vi "wmlf Defects Script.vi"(0 "File Path":path, 2 "threshoulds":dbl[](array[numeric])=[900.0, 900.0, 1000.0, 1200.0, 1800.0, 1800.0, 2000.0, 2400.0], 3 "margin":dbl[](array[numeric]), 5 "Image 3":T1(plugin-control), 7 "error in (no error)":errorcluster) -> (18 "function return":i32, 20 "x-y defects locs":dbl[][](array[numeric]), 21 "defnum":dbl, 22 "def type":dbl, 23 "frame situation":dbl, 24 "obj num":dbl, 25 "def ratio":dbl, 26 "crop array":dbl[][](array[numeric]), 27 "error out":errorcluster)   [LabVIEW 2019, in "defectsWrapper.lvlib"]
doc: "int wmlfDefectsScript(double* c2dArray, double* d2dArray, double* e2dArray ,double* f2dArray, double* g2dArray,\n double* h2dArray , double* i2dArray, double* j2dArray,double* k2dArray, double* l2dArray, int numRows, int numColumns,\n int Rows, int Columns, int Rows1, int Columns1, int Rows2, int Columns2, int Rows3, int Columns3,\n int Rows4, int Columns4,int Rows5, int Columns5,int Rows6, int Columns6, int Rows7, int Columns7,\n int Rows8, int Columns8 );"
uses:
  defectsWrapper.lvlib
  defectsWrapper.dll
panel:
  out "x array":dbl[](array[numeric])
  out "ydef":dbl[][](array[numeric])
  out "xdef":dbl[][](array[numeric])
  out "initialized array":dbl[][](array[numeric])
  out "Image 2":T1(plugin-control)
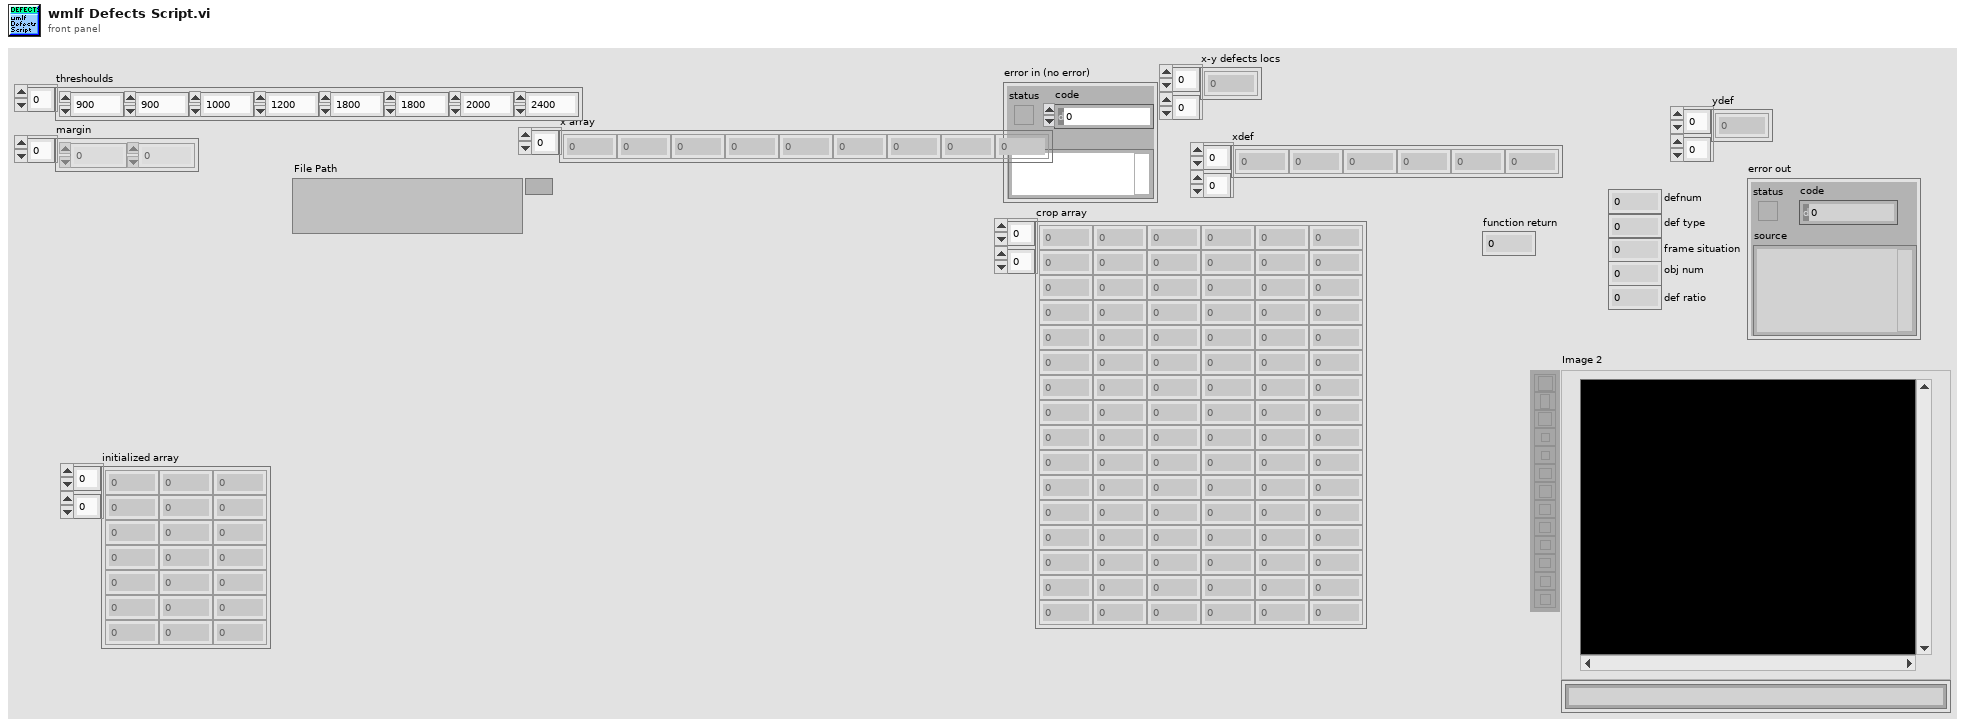
[diagram p1: front panel]
types:
  T1 = typedef "IMAQ Image.ctl" = refnum<image>
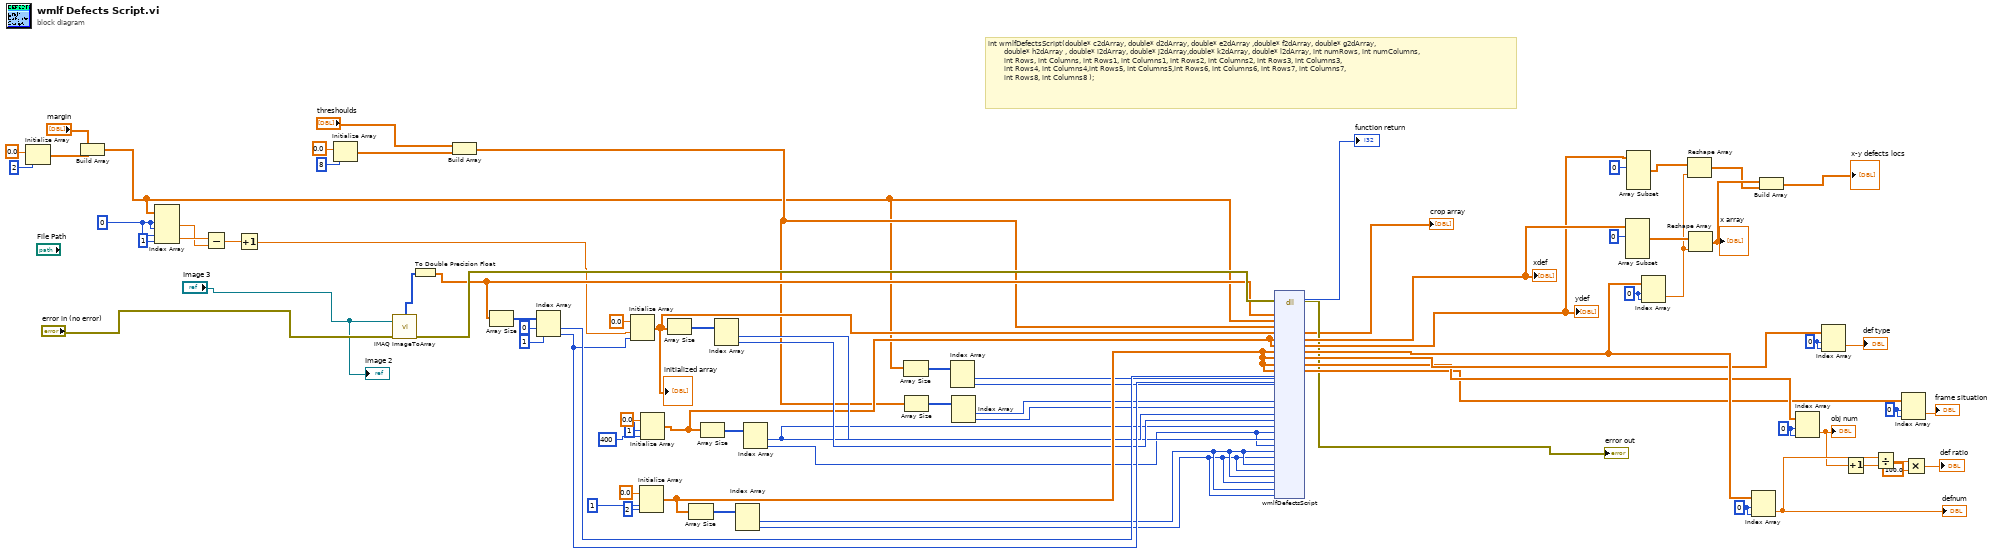
[diagram p0: block diagram]
diagram:
  w24 = 0 ("index (row)")
  w26 = 0 ("index (row)")
  w29 = 0 ("index (row)")
  w30 = 0 ("index (row)")
  w38 = 0 ("index (row)")
  w45 = 0 ("index (row)")
  # "int wmlfDefectsScript(double* c2dArray, double* d2dArray, double* e2dArray ,double* f2dArray, double* g2dArray,\n        double* h2dArray , double* i2dArray, double* j2dArray,double* k2dArray, double* l2dArray, int numRows, int numColumns,\n        int Rows, int Columns, int Rows1, int Columns1, int Rows2, int Columns2, int Rows3, int Columns3,\n        int Rows4, int Columns4,int Rows5, int Columns5,int Rows6, int Columns6, int Rows7, int Columns7,\n        int Rows8, int Columns8 );"
  n1 = Initialize Array(0.0 ("element"), 2 ("dimension size")) -> (w10:dbl[])
  n2 = Build Array("margin", w10) -> (w8:dbl[][])
  n3 = Index Array(array=w8, index (row) #1=w38, index (col) #1=w38, index (row) #2=w38, index (col) #2=1 ("disabled index (col)")) -> (element #1=w35:dbl, element #2=w36:dbl)
  n4 = Subtract(x=w36, y=w35) -> (x-y=w34:dbl)
  n5 = Increment(x=w34) -> (x+1=w33:dbl)
  n6 = Initialize Array(0.0 ("element"), 8 ("dimension size")) -> (w15:dbl[])
  n7 = call "IMAQ ImageToArray"("error in (no error)"="error in (no error)", "Image"="Image 3") -> ("error out"=w67:errorcluster, "Image Pixels (U8)"=w79:u8[][])  [unwired: 2 in, 3 out]
  n8 = To Double Precision Float(number=w79) -> (double precision float=w66:dbl[][])
  n9 = Build Array("threshoulds", w15) -> (w13:dbl[][])
  n10 = Array Size(array=w66) -> (size(s)=w80:i32[])
  n11 = Index Array(array=w80, index #1=0 ("index"), index #2=1 ("index")) -> (element #1=w63:i32, element #2=w62:i32)
  n12 = Initialize Array(0.0 ("element"), w33, w62) -> (w65:dbl[][])
  "initialized array" <- w65
  n13 = Initialize Array(0.0 ("element"), 1 ("dimension size"), 2 ("dimension size")) -> (w64:dbl[][])
  n14 = Initialize Array(0.0 ("element"), 1 ("dimension size"), 400 ("dimension size")) -> (w32:dbl[][])
  n15 = Array Size(array=w65) -> (size(s)=w77:i32[])
  n16 = Array Size(array=w64) -> (size(s)=w68:i32[])
  n17 = Array Size(array=w32) -> (size(s)=w51:i32[])
  n18 = Index Array(array=w77) -> (element #1=w57:i32, element #2=w56:i32)  [unwired: 2 in]
  n19 = Index Array(array=w68) -> (element #1=w55:i32, element #2=w54:i32)  [unwired: 2 in]
  n20 = Index Array(array=w51) -> (element #1=w50:i32, element #2=w49:i32)  [unwired: 2 in]
  n21 = Array Size(array=w8) -> (size(s)=w70:i32[])
  n22 = Array Size(array=w13) -> (size(s)=w69:i32[])
  n23 = Index Array(array=w70) -> (element #1=w61:i32, element #2=w60:i32)  [unwired: 2 in]
  n24 = Index Array(array=w69) -> (element #1=w59:i32, element #2=w58:i32)  [unwired: 2 in]
  n25 = dll-call lib="C:/Users/user/Desktop/defectsWrapper/defectsWrapper.*" fn="wmlfDefectsScript"(error in=w67, "c2dArray"=w66, "d2dArray"=w8, "e2dArray"=w13, "f2dArray"=w65, "g2dArray"=w32, "h2dArray"=w32, "i2dArray"=w64, "j2dArray"=w64, "k2dArray"=w64, "l2dArray"=w64, "numRows"=w63, "numColumns"=w62, "Rows"=w61, "Columns"=w60, "Rows1"=w59, "Columns1"=w58, "Rows2"=w57, "Columns2"=w56, "Rows3"=w50, "Columns3"=w49, "Rows4"=w50, "Columns4"=w49, "Rows5"=w55, "Columns5"=w54, "Rows6"=w55, "Columns6"=w54, "Rows7"=w55, "Columns7"=w54, "Rows8"=w55, "Columns8"=w54) -> (error out=→"error out":errorcluster, "return type"=→"function return":i32, "f2dArray"=→"crop array":dbl[][], "g2dArray"=w48:dbl[][], "h2dArray"=w43:dbl[][], "i2dArray"=w31:dbl[][], "j2dArray"=w28:dbl[][], "k2dArray"=w25:dbl[][], "l2dArray"=w23:dbl[][])  [unwired: 25 in, 1 out]
  "xdef" <- w48
  "ydef" <- w43
  n26 = Array Subset(array=w48, index (row)=0 ("index")) -> (w46:dbl[][])  [unwired: 3 in]
  n27 = Array Subset(array=w43, index (row)=0 ("index")) -> (w42:dbl[][])  [unwired: 3 in]
  n28 = Index Array(array=w31, index (row)=w45, index (col)=w45) -> (element=w41:dbl)
  n29 = Reshape Array(w42, w41) -> (w39:dbl[])
  n30 = Reshape Array(w46, w41) -> (w40:dbl[])
  "x array" <- w40
  n31 = Index Array(array=w31, index (row)=w30, index (col)=w30) -> (element=w21:dbl)
  "defnum" <- w21
  n32 = Build Array(w40, w39) -> (→"x-y defects locs":dbl[][])
  n33 = Index Array(array=w25, index (row)=w26, index (col)=w26) -> (element=w2:dbl)
  "obj num" <- w2
  n34 = Index Array(array=w28, index (row)=w29, index (col)=w29) -> (element=→"def type":dbl)
  n35 = Increment(x=w2) -> (x+1=w1:dbl)
  n36 = Divide(x=w21, y=w1) -> (x/y=w20:dbl)
  n37 = Index Array(array=w23, index (row)=w24, index (col)=w24) -> (element=→"frame situation":dbl)
  n38 = Multiply(x=w20, y=100.0) -> (x*y=→"def ratio":dbl)
  "Image 2" <- "Image 3"
